vi "PH_Cam_BaseClass.ProcCases.vi"(0 "i ref in":refnum<vi>, 1 "selector":string, 2 "data":T1, 3 "call cluster":T2={"Object"="", "Selector"="", "CallType"=enum."synchronous", "Async Object"="", "Async Selector"="", "Data Descriptor"="", "Data"=[], "Error #"=0, "Expire"=0}, 5 "error in":errorcluster) -> (14 "i ref out":refnum<vi>, 17 "answer cluster":T2={"Object"="", "Selector"="", "CallType"=enum."synchronous", "Async Object"="", "Async Selector"="", "Data Descriptor"="", "Data"=[], "Error #"=0, "Expire"=0}, 19 "error out":errorcluster)   [LabVIEW 2014, in "PH_Cam_BaseClass.lvlib"]
doc: "This method is called by a process from within the default case in the event loop. The methods of a class that are linked to events will be called from THIS method. Add your code here."
uses:
  PH_Cam_BaseClass.lvlib
  CSCore/CSSystem/CoreDefs/CoreDefs.call_type.ctl
  CSCore/BaseProcess/BaseProcess.descriptor string definition.ctl
  CSCore/CSSystem/CoreDefs/CoreDefs.rawDataType.ctl
  CSCore/CSSystem/CoreLib/CoreLib.string 2 byte array.vi
  CSCore/CSSystem/CoreLib/CoreLib.byte array 2 string.vi
  CSCore/CSSystem/CoreLib/CoreLib.byte array 2 short.vi
  CSCore/CSSystem/CoreLib/CoreLib.byte array 2 double.vi
  CSCore/CSSystem/CoreLib/CoreLib.byte array 2 int.vi
  CSCore/CSSystem/CoreLib/CoreLib.lvlib
  CSCore/BaseProcess/BaseProcess.lvlib
  PH_Common/PH_Common.lvlib
  PH_PSDBWriter/PH_PSDBWriter.lvlib
panel:
  in  "EP":cluster{"Red":u8, "Green":u8, "Blue":u8}[](array[cluster])=[{"Red"=0, "Green"=255, "Blue"=0}, {"Red"=0, "Green"=245, "Blue"=0}, {"Red"=0, "Green"=235, "Blue"=0}, {"Red"=0, "Green"=225, "Blue"=0}, {"Red"=0, "Green"=215, "Blue"=0}, {"Red"=0, "Green"=205, "Blue"=0}, {"Red"=0, "Green"=195, "Blue"=0}, {"Red"=0, "Green"=185, "Blue"=0}, {"Red"=0, "Green"=175, "Blue"=0}, {"Red"=0, "Green"=165, "Blue"=0}, {"Red"=10, "Green"=10, "Blue"=10}, {"Red"=11, "Green"=11, "Blue"=11}, {"Red"=12, "Green"=12, "Blue"=12}, {"Red"=13, "Green"=13, "Blue"=13}, {"Red"=14, "Green"=14, "Blue"=14}, {"Red"=15, "Green"=15, "Blue"=15}, {"Red"=16, "Green"=16, "Blue"=16}, {"Red"=17, "Green"=17, "Blue"=17}, {"Red"=18, "Green"=18, "Blue"=18}, {"Red"=19, "Green"=19, "Blue"=19}, {"Red"=20, "Green"=20, "Blue"=20}, {"Red"=21, "Green"=21, "Blue"=21}, {"Red"=22, "Green"=22, "Blue"=22}, {"Red"=23, "Green"=23, "Blue"=23}, {"Red"=24, "Green"=24, "Blue"=24}, {"Red"=25, "Green"=25, "Blue"=25}, {"Red"=26, "Green"=26, "Blue"=26}, {"Red"=27, "Green"=27, "Blue"=27}, {"Red"=28, "Green"=28, "Blue"=28}, {"Red"=29, "Green"=29, "Blue"=29}, {"Red"=30, "Green"=30, "Blue"=30}, {"Red"=31, "Green"=31, "Blue"=31}, {"Red"=32, "Green"=32, "Blue"=32}, {"Red"=33, "Green"=33, "Blue"=33}, {"Red"=34, "Green"=34, "Blue"=34}, {"Red"=35, "Green"=35, "Blue"=35}, {"Red"=36, "Green"=36, "Blue"=36}, {"Red"=37, "Green"=37, "Blue"=37}, {"Red"=38, "Green"=38, "Blue"=38}, {"Red"=39, "Green"=39, "Blue"=39}, {"Red"=40, "Green"=40, "Blue"=40}, {"Red"=41, "Green"=41, "Blue"=41}, {"Red"=42, "Green"=42, "Blue"=42}, {"Red"=43, "Green"=43, "Blue"=43}, {"Red"=44, "Green"=44, "Blue"=44}, {"Red"=45, "Green"=45, "Blue"=45}, {"Red"=46, "Green"=46, "Blue"=46}, {"Red"=47, "Green"=47, "Blue"=47}, {"Red"=48, "Green"=48, "Blue"=48}, {"Red"=49, "Green"=49, "Blue"=49}, {"Red"=50, "Green"=50, "Blue"=50}, {"Red"=51, "Green"=51, "Blue"=51}, {"Red"=52, "Green"=52, "Blue"=52}, {"Red"=53, "Green"=53, "Blue"=53}, {"Red"=54, "Green"=54, "Blue"=54}, {"Red"=55, "Green"=55, "Blue"=55}, {"Red"=56, "Green"=56, "Blue"=56}, {"Red"=57, "Green"=57, "Blue"=57}, {"Red"=58, "Green"=58, "Blue"=58}, {"Red"=59, "Green"=59, "Blue"=59}, {"Red"=60, "Green"=60, "Blue"=60}, {"Red"=61, "Green"=61, "Blue"=61}, {"Red"=62, "Green"=62, "Blue"=62}, {"Red"=63, "Green"=63, "Blue"=63}, {"Red"=64, "Green"=64, "Blue"=64}, {"Red"=65, "Green"=65, "Blue"=65}, {"Red"=66, "Green"=66, "Blue"=66}, {"Red"=67, "Green"=67, "Blue"=67}, {"Red"=68, "Green"=68, "Blue"=68}, {"Red"=69, "Green"=69, "Blue"=69}, {"Red"=70, "Green"=70, "Blue"=70}, {"Red"=71, "Green"=71, "Blue"=71}, {"Red"=72, "Green"=72, "Blue"=72}, {"Red"=73, "Green"=73, "Blue"=73}, {"Red"=74, "Green"=74, "Blue"=74}, {"Red"=75, "Green"=75, "Blue"=75}, {"Red"=76, "Green"=76, "Blue"=76}, {"Red"=77, "Green"=77, "Blue"=77}, {"Red"=78, "Green"=78, "Blue"=78}, {"Red"=79, "Green"=79, "Blue"=79}, {"Red"=80, "Green"=80, "Blue"=80}, {"Red"=81, "Green"=81, "Blue"=81}, {"Red"=82, "Green"=82, "Blue"=82}, {"Red"=83, "Green"=83, "Blue"=83}, {"Red"=84, "Green"=84, "Blue"=84}, {"Red"=85, "Green"=85, "Blue"=85}, {"Red"=86, "Green"=86, "Blue"=86}, {"Red"=87, "Green"=87, "Blue"=87}, {"Red"=88, "Green"=88, "Blue"=88}, {"Red"=89, "Green"=89, "Blue"=89}, {"Red"=90, "Green"=90, "Blue"=90}, {"Red"=91, "Green"=91, "Blue"=91}, {"Red"=92, "Green"=92, "Blue"=92}, {"Red"=93, "Green"=93, "Blue"=93}, {"Red"=94, "Green"=94, "Blue"=94}, {"Red"=95, "Green"=95, "Blue"=95}, {"Red"=96, "Green"=96, "Blue"=96}, {"Red"=97, "Green"=97, "Blue"=97}, {"Red"=98, "Green"=98, "Blue"=98}, {"Red"=99, "Green"=99, "Blue"=99}, {"Red"=100, "Green"=100, "Blue"=100}, {"Red"=101, "Green"=101, "Blue"=101}, {"Red"=102, "Green"=102, "Blue"=102}, {"Red"=103, "Green"=103, "Blue"=103}, {"Red"=104, "Green"=104, "Blue"=104}, {"Red"=105, "Green"=105, "Blue"=105}, {"Red"=106, "Green"=106, "Blue"=106}, {"Red"=107, "Green"=107, "Blue"=107}, {"Red"=108, "Green"=108, "Blue"=108}, {"Red"=109, "Green"=109, "Blue"=109}, {"Red"=110, "Green"=110, "Blue"=110}, {"Red"=111, "Green"=111, "Blue"=111}, {"Red"=112, "Green"=112, "Blue"=112}, {"Red"=113, "Green"=113, "Blue"=113}, {"Red"=114, "Green"=114, "Blue"=114}, {"Red"=115, "Green"=115, "Blue"=115}, {"Red"=116, "Green"=116, "Blue"=116}, {"Red"=117, "Green"=117, "Blue"=117}, {"Red"=118, "Green"=118, "Blue"=118}, {"Red"=119, "Green"=119, "Blue"=119}, {"Red"=120, "Green"=120, "Blue"=120}, {"Red"=121, "Green"=121, "Blue"=121}, {"Red"=122, "Green"=122, "Blue"=122}, {"Red"=123, "Green"=123, "Blue"=123}, {"Red"=124, "Green"=124, "Blue"=124}, {"Red"=125, "Green"=125, "Blue"=125}, {"Red"=126, "Green"=126, "Blue"=126}, {"Red"=127, "Green"=127, "Blue"=127}, {"Red"=128, "Green"=128, "Blue"=128}, {"Red"=129, "Green"=129, "Blue"=129}, {"Red"=130, "Green"=130, "Blue"=130}, {"Red"=131, "Green"=131, "Blue"=131}, {"Red"=132, "Green"=132, "Blue"=132}, {"Red"=133, "Green"=133, "Blue"=133}, {"Red"=134, "Green"=134, "Blue"=134}, {"Red"=135, "Green"=135, "Blue"=135}, {"Red"=136, "Green"=136, "Blue"=136}, {"Red"=137, "Green"=137, "Blue"=137}, {"Red"=138, "Green"=138, "Blue"=138}, {"Red"=139, "Green"=139, "Blue"=139}, {"Red"=140, "Green"=140, "Blue"=140}, {"Red"=141, "Green"=141, "Blue"=141}, {"Red"=142, "Green"=142, "Blue"=142}, {"Red"=143, "Green"=143, "Blue"=143}, {"Red"=144, "Green"=144, "Blue"=144}, {"Red"=145, "Green"=145, "Blue"=145}, {"Red"=146, "Green"=146, "Blue"=146}, {"Red"=147, "Green"=147, "Blue"=147}, {"Red"=148, "Green"=148, "Blue"=148}, {"Red"=149, "Green"=149, "Blue"=149}, {"Red"=150, "Green"=150, "Blue"=150}, {"Red"=151, "Green"=151, "Blue"=151}, {"Red"=152, "Green"=152, "Blue"=152}, {"Red"=153, "Green"=153, "Blue"=153}, {"Red"=154, "Green"=154, "Blue"=154}, {"Red"=155, "Green"=155, "Blue"=155}, {"Red"=156, "Green"=156, "Blue"=156}, {"Red"=157, "Green"=157, "Blue"=157}, {"Red"=158, "Green"=158, "Blue"=158}, {"Red"=159, "Green"=159, "Blue"=159}, {"Red"=160, "Green"=160, "Blue"=160}, {"Red"=161, "Green"=161, "Blue"=161}, {"Red"=162, "Green"=162, "Blue"=162}, {"Red"=163, "Green"=163, "Blue"=163}, {"Red"=164, "Green"=164, "Blue"=164}, {"Red"=165, "Green"=165, "Blue"=165}, {"Red"=166, "Green"=166, "Blue"=166}, {"Red"=167, "Green"=167, "Blue"=167}, {"Red"=168, "Green"=168, "Blue"=168}, {"Red"=169, "Green"=169, "Blue"=169}, {"Red"=170, "Green"=170, "Blue"=170}, {"Red"=171, "Green"=171, "Blue"=171}, {"Red"=172, "Green"=172, "Blue"=172}, {"Red"=173, "Green"=173, "Blue"=173}, {"Red"=174, "Green"=174, "Blue"=174}, {"Red"=175, "Green"=175, "Blue"=175}, {"Red"=176, "Green"=176, "Blue"=176}, {"Red"=177, "Green"=177, "Blue"=177}, {"Red"=178, "Green"=178, "Blue"=178}, {"Red"=179, "Green"=179, "Blue"=179}, {"Red"=180, "Green"=180, "Blue"=180}, {"Red"=181, "Green"=181, "Blue"=181}, {"Red"=182, "Green"=182, "Blue"=182}, {"Red"=183, "Green"=183, "Blue"=183}, {"Red"=184, "Green"=184, "Blue"=184}, {"Red"=185, "Green"=185, "Blue"=185}, {"Red"=186, "Green"=186, "Blue"=186}, {"Red"=187, "Green"=187, "Blue"=187}, {"Red"=188, "Green"=188, "Blue"=188}, {"Red"=189, "Green"=189, "Blue"=189}, {"Red"=190, "Green"=190, "Blue"=190}, {"Red"=191, "Green"=191, "Blue"=191}, {"Red"=192, "Green"=192, "Blue"=192}, {"Red"=193, "Green"=193, "Blue"=193}, {"Red"=194, "Green"=194, "Blue"=194}, {"Red"=195, "Green"=195, "Blue"=195}, {"Red"=196, "Green"=196, "Blue"=196}, {"Red"=197, "Green"=197, "Blue"=197}, {"Red"=198, "Green"=198, "Blue"=198}, {"Red"=199, "Green"=199, "Blue"=199}, {"Red"=200, "Green"=200, "Blue"=200}, {"Red"=201, "Green"=201, "Blue"=201}, {"Red"=202, "Green"=202, "Blue"=202}, {"Red"=203, "Green"=203, "Blue"=203}, {"Red"=204, "Green"=204, "Blue"=204}, {"Red"=205, "Green"=205, "Blue"=205}, {"Red"=206, "Green"=206, "Blue"=206}, {"Red"=207, "Green"=207, "Blue"=207}, {"Red"=208, "Green"=208, "Blue"=208}, {"Red"=209, "Green"=209, "Blue"=209}, {"Red"=210, "Green"=210, "Blue"=210}, {"Red"=211, "Green"=211, "Blue"=211}, {"Red"=212, "Green"=212, "Blue"=212}, {"Red"=213, "Green"=213, "Blue"=213}, {"Red"=214, "Green"=214, "Blue"=214}, {"Red"=215, "Green"=215, "Blue"=215}, {"Red"=216, "Green"=216, "Blue"=216}, {"Red"=217, "Green"=217, "Blue"=217}, {"Red"=218, "Green"=218, "Blue"=218}, {"Red"=219, "Green"=219, "Blue"=219}, {"Red"=220, "Green"=220, "Blue"=220}, {"Red"=221, "Green"=221, "Blue"=221}, {"Red"=222, "Green"=222, "Blue"=222}, {"Red"=223, "Green"=223, "Blue"=223}, {"Red"=224, "Green"=224, "Blue"=224}, {"Red"=225, "Green"=225, "Blue"=225}, {"Red"=226, "Green"=226, "Blue"=226}, {"Red"=227, "Green"=227, "Blue"=227}, {"Red"=228, "Green"=228, "Blue"=228}, {"Red"=229, "Green"=229, "Blue"=229}, {"Red"=230, "Green"=230, "Blue"=230}, {"Red"=231, "Green"=231, "Blue"=231}, {"Red"=232, "Green"=232, "Blue"=232}, {"Red"=233, "Green"=233, "Blue"=233}, {"Red"=234, "Green"=234, "Blue"=234}, {"Red"=235, "Green"=235, "Blue"=235}, {"Red"=236, "Green"=236, "Blue"=236}, {"Red"=237, "Green"=237, "Blue"=237}, {"Red"=238, "Green"=238, "Blue"=238}, {"Red"=239, "Green"=239, "Blue"=239}, {"Red"=240, "Green"=240, "Blue"=240}, {"Red"=241, "Green"=241, "Blue"=241}, {"Red"=242, "Green"=242, "Blue"=242}, {"Red"=243, "Green"=243, "Blue"=243}, {"Red"=244, "Green"=244, "Blue"=244}, {"Red"=245, "Green"=245, "Blue"=245}, {"Red"=165, "Green"=0, "Blue"=0}, {"Red"=175, "Green"=0, "Blue"=0}, {"Red"=185, "Green"=0, "Blue"=0}, {"Red"=195, "Green"=0, "Blue"=0}, {"Red"=205, "Green"=0, "Blue"=0}, {"Red"=215, "Green"=0, "Blue"=0}, {"Red"=225, "Green"=0, "Blue"=0}, {"Red"=235, "Green"=0, "Blue"=0}, {"Red"=245, "Green"=0, "Blue"=0}, {"Red"=255, "Green"=0, "Blue"=0}]
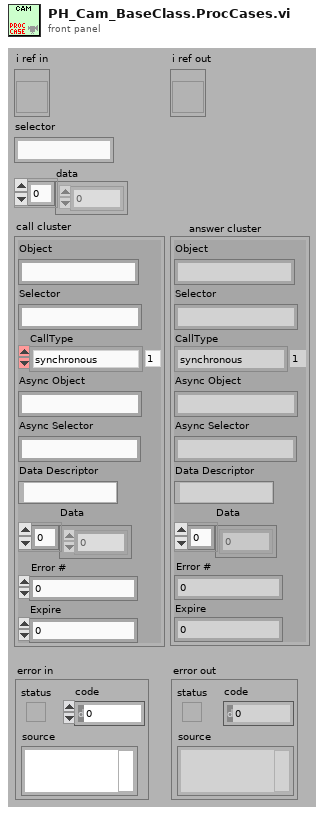
[diagram p1: front panel]
types:
  T1 = typedef "CoreDefs.rawDataType.ctl" = i8[]
  T2 = typedef "CoreDefs.call_type.ctl" = cluster{"Object":string, "Selector":string, "CallType":enum16{"simple", "synchronous", "asynchronous"}, "Async Object":string, "Async Selector":string, "Data Descriptor":T3, "Data":T1, "Error #":i32, "Expire":u32}
  T3 = typedef "BaseProcess.lvlib/BaseProcess.descriptor string definition.ctl" = string
  T4 = typedef "PH_Cam_BaseClass.lvlib/PH_Cam_BaseClass.i attribute.ctl" = cluster{"Gui Refs":T5, "Cam":cluster{"Source Notifier":refnum<notifier>, "Error":errorcluster, "Camera ID":string}, "Images":cluster{"Cam":T6, "Operation":T6, "PSDB":T6}, "Window Image":cluster{"Indicate Image":bool, "Window No.":i32, "Scale Facor":dbl, "Center Cross":bool, "Subtract Backgr":bool, "CoG":bool, "Color Palette":cluster{"Red":u8, "Green":u8, "Blue":u8}[], "Image On":bool}, "Default Prdc Int":i32, "Performance":cluster{"on":bool, "Timestamp Last Frame":i32}, "Histogram":cluster{"on":bool, "Mapping":bool}, "Save Image":cluster{"Save":bool, "File refnum":refnum<file>}, "Setting Service ID":i32, "Screen":cluster{"x-resolution":i16, "y-resolution":i16}, "On":bool, "Constructor finished":bool, "configured":bool}
  T5 = typedef "PH_Cam_BaseClass.lvlib/PH_Cam_BaseClass.GUI Refs.ctl" = cluster{"Frame Rate":refnum<vi>, "Get Frame Rate":refnum<vi>, "Show Image":refnum<vi>, "Get Histogram":refnum<vi>, "Mapping":refnum<vi>, "Histogram":refnum<vi>, "Center Cross":refnum<vi>, "Center of Gravity":refnum<vi>, "Scale Factor [%]":refnum<vi>, "Save Image":refnum<vi>, "Palette":refnum<vi>, "Subtract Background":refnum<vi>, "Cam Error":refnum<vi>, "On":refnum<vi>, "Cam List":refnum<vi>}
  T6 = typedef "IMAQ Image.ctl" = refnum<image>
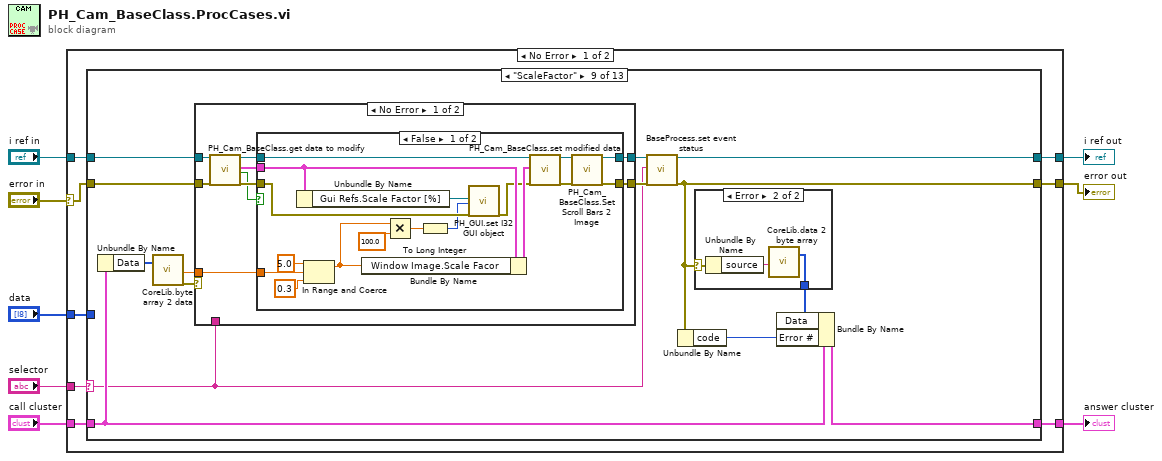
[diagram p0: block diagram]
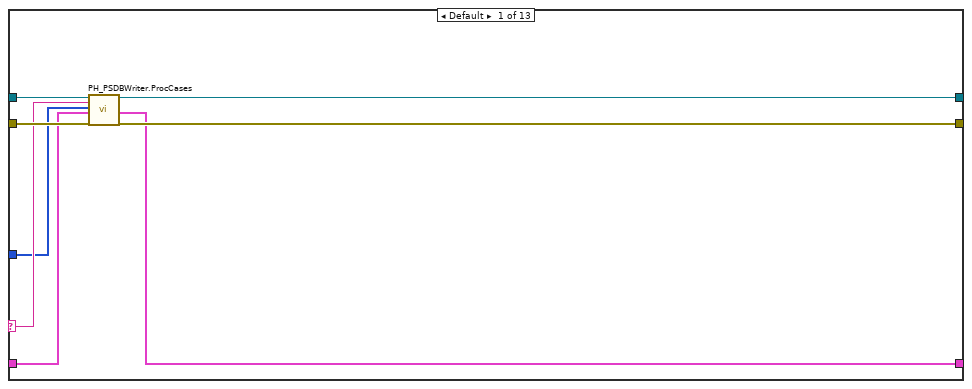
[diagram p2: hidden frame]
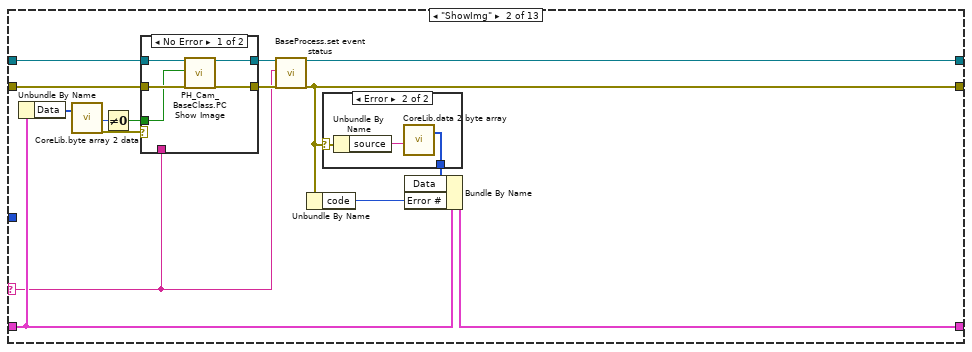
[diagram p3: hidden frame]
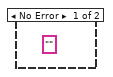
[diagram p4: hidden frame]
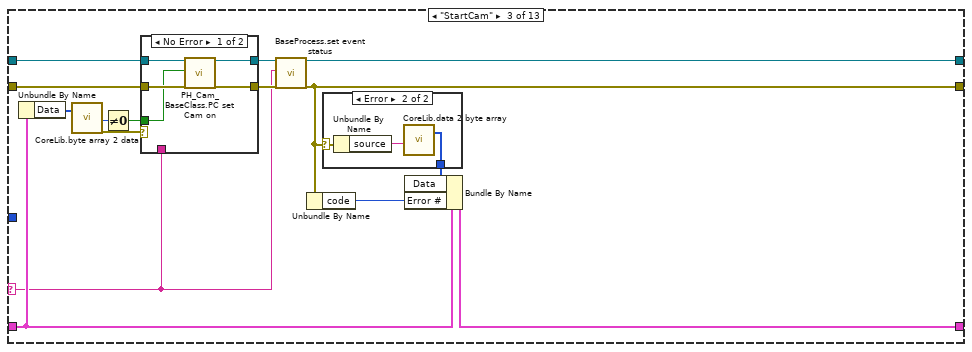
[diagram p6: hidden frame]
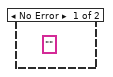
[diagram p7: hidden frame]
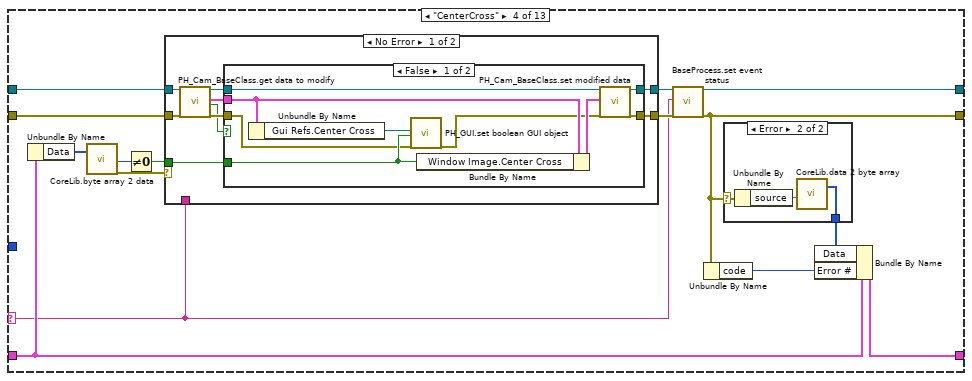
[diagram p9: hidden frame]
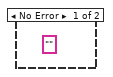
[diagram p10: hidden frame]
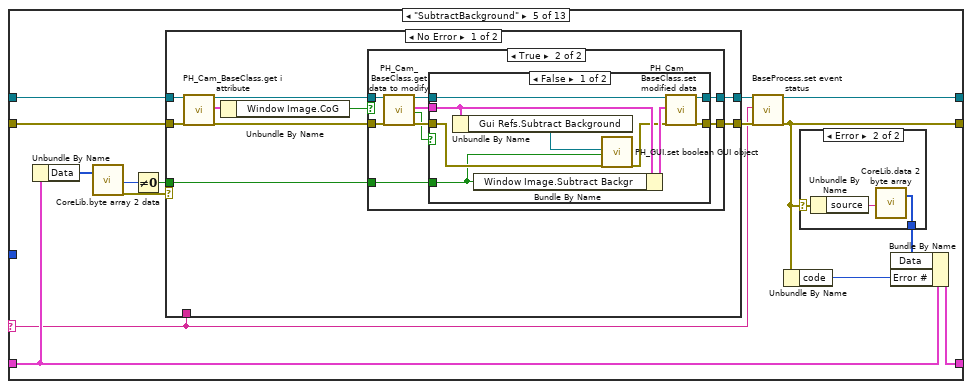
[diagram p13: hidden frame]
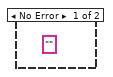
[diagram p14: hidden frame]
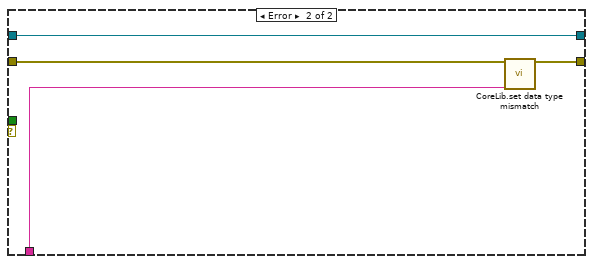
[diagram p17: hidden frame]
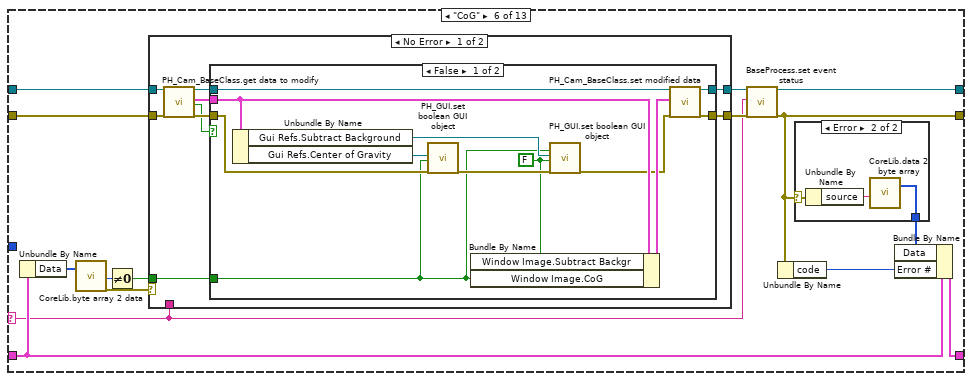
[diagram p18: hidden frame]
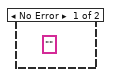
[diagram p19: hidden frame]
diagram:
  n1 = case shown="No Error" "error in" {
    selector: "error in" -> [w9 w553]
    tunnel: "selector" -> [w16 _]
    tunnel: [w15 w552] -> w7
    tunnel: "call cluster" -> [w14 w552]
    tunnel: "i ref in" -> [w13 w554]
    tunnel: [w12 w554] -> w4
    tunnel: [w11 w553] -> w3
    tunnel: "data" -> [w10 _]
    frame No Error {
      n2 = case shown="\"ScaleFactor\"" w16 {
        selector: w16 -> [w19 w31 w58 w85 w127 w180 w234 w283 w338 w388 w439 w492 w513]
        tunnel: w13 -> [w18 w39 w66 w93 w135 w188 w242 w291 w346 w396 w447 w500 w518]
        tunnel: [w24 w30 w57 w84 w126 w179 w233 w282 w337 w387 w438 w491 w523] -> w12
        tunnel: w14 -> [w20 w36 w63 w90 w132 w185 w239 w288 w343 w393 w444 w497 w516]
        tunnel: [w21 w35 w62 w89 w131 w184 w238 w287 w342 w392 w443 w496 w525] -> w15
        tunnel: w9 -> [w23 w38 w65 w92 w134 w187 w241 w290 w345 w395 w446 w499 w517]
        tunnel: [w22 w32 w59 w86 w128 w181 w235 w284 w339 w389 w440 w493 w524] -> w11
        tunnel: w10 -> [w17 _ _ _ _ _ _ _ _ _ _ _ _]
        frame Default {
          # "In the default case, always call the ProcCase method of the parent class"
          n3 = call "PH_PSDBWriter.ProcCases.vi"("i ref in"=w18, "selector"=w19, "Data"=w17, "call cluster"=w20, "error in"=w23) -> ("i ref out"=w24:refnum<vi>, "answer cluster"=w21:T2, "error out"=w22:errorcluster)  [unwired: 12 in]
        }
        frame "ShowImg" {
          n4 = Unbundle By Name(w36) -> ("Data"=w26:T1)
          n5 = call-poly "CoreLib.byte array 2 data.vi"("byteArray"=w26) -> ("i16"=w29:i16, "error out"=w28:errorcluster)  [unwired: 16 in, 1 out]
          n6 = Not Equal To 0?(x=w29) -> (x != 0?=w27:bool)
          n7 = case shown="No Error" w28 {
            tunnel: [w44 w51] -> w34
            tunnel: w39 -> [w46 w51]
            tunnel: w38 -> [w47 w50]
            tunnel: [w43 w49] -> w33
            tunnel: w31 -> [_ w48]
            tunnel: w27 -> [w45 _]
            frame No Error {
              n8 = call "PH_Cam_BaseClass.PC Show Image.vi"("i ref in"=w46, "Show Image"=w45, "error IO"=w47) -> ("i ref out"=w44:refnum<vi>, "error out"=w43:errorcluster)  [unwired: 15 in]
            }
            frame Error {
              n9 = call "CoreLib.set data type mismatch.vi"("error in (no error)"=w50, "error source"=w48) -> ("error out"=w49:errorcluster)  [unwired: 17 in]
            }
          }
          n10 = call "BaseProcess.set event status.vi"("i ref in"=w34, "EventStatus"=w31, "error in (no error)"=w33) -> ("i ref out"=w30:refnum<vi>, "error out"=w32:errorcluster)  [unwired: 14 in, 1 out]
          n11 = Unbundle By Name(w32) -> ("code"=w37:i32)
          n12 = case shown="Error" w32 {
            selector: w32 -> [_ w42]
            tunnel: [_ w40] -> w25
            frame No Error {
              (unwired) "" ("source")
            }
            frame Error {
              n13 = Unbundle By Name(w42) -> ("source"=w41:string)
              n14 = call-poly "CoreLib.data 2 byte array.vi"("string"=w41) -> ("byteArray out"=w40:T1)  [unwired: 18 in]
            }
          }
          n15 = Bundle By Name(cluster=w36, "Data"=w25, "Error #"=w37) -> (w35:T2)
        }
        frame "StartCam" {
          n16 = Unbundle By Name(w63) -> ("Data"=w53:T1)
          n17 = call-poly "CoreLib.byte array 2 data.vi"("byteArray"=w53) -> ("i16"=w56:i16, "error out"=w55:errorcluster)  [unwired: 16 in, 1 out]
          n18 = Not Equal To 0?(x=w56) -> (x != 0?=w54:bool)
          n19 = case shown="No Error" w55 {
            tunnel: [w71 w78] -> w61
            tunnel: w66 -> [w73 w78]
            tunnel: w65 -> [w74 w77]
            tunnel: [w70 w76] -> w60
            tunnel: w58 -> [_ w75]
            tunnel: w54 -> [w72 _]
            frame No Error {
              n20 = call "PH_Cam_BaseClass.PC set Cam on.vi"("i ref in"=w73, "Cam on"=w72, "error in (no error)"=w74) -> ("i ref out"=w71:refnum<vi>, "error out"=w70:errorcluster)  [unwired: 15 in]
            }
            frame Error {
              n21 = call "CoreLib.set data type mismatch.vi"("error in (no error)"=w77, "error source"=w75) -> ("error out"=w76:errorcluster)  [unwired: 17 in]
            }
          }
          n22 = call "BaseProcess.set event status.vi"("i ref in"=w61, "EventStatus"=w58, "error in (no error)"=w60) -> ("i ref out"=w57:refnum<vi>, "error out"=w59:errorcluster)  [unwired: 14 in, 1 out]
          n23 = Unbundle By Name(w59) -> ("code"=w64:i32)
          n24 = case shown="Error" w59 {
            selector: w59 -> [_ w69]
            tunnel: [_ w67] -> w52
            frame No Error {
              (unwired) "" ("source")
            }
            frame Error {
              n25 = Unbundle By Name(w69) -> ("source"=w68:string)
              n26 = call-poly "CoreLib.data 2 byte array.vi"("string"=w68) -> ("byteArray out"=w67:T1)  [unwired: 18 in]
            }
          }
          n27 = Bundle By Name(cluster=w63, "Data"=w52, "Error #"=w64) -> (w62:T2)
        }
        frame "CenterCross" {
          n28 = Unbundle By Name(w90) -> ("Data"=w80:T1)
          n29 = call-poly "CoreLib.byte array 2 data.vi"("byteArray"=w80) -> ("i16"=w83:i16, "error out"=w81:errorcluster)  [unwired: 16 in, 1 out]
          n30 = Not Equal To 0?(x=w83) -> (x != 0?=w82:bool)
          n31 = case shown="No Error" w81 {
            tunnel: [w100 w120] -> w88
            tunnel: w93 -> [w104 w120]
            tunnel: w92 -> [w105 w119]
            tunnel: [w102 w118] -> w87
            tunnel: w85 -> [_ w117]
            tunnel: w82 -> [w98 _]
            frame No Error {
              n32 = call "PH_Cam_BaseClass.get data to modify.vi"("i ref in"=w104, "error in (no error)"=w105) -> ("i ref out"=w101:refnum<vi>, "i attribute"=w99:T4, "timed out"=w97:bool, "error out"=w103:errorcluster)  [unwired: 14 in]
              n33 = case shown="False" w97 {
                tunnel: w103 -> [w107 w115]
                tunnel: [w114 w115] -> w102
                tunnel: w101 -> [w113 w116]
                tunnel: [w112 w116] -> w100
                tunnel: w99 -> [w110 _]
                tunnel: w98 -> [w108 _]
                frame False {
                  n34 = Unbundle By Name(w110) -> ("Gui Refs.Center Cross"=w109:refnum<vi>)
                  n35 = call "PH_GUI.set boolean GUI object.vi"("Boolean Knob GUI Ref"=w109, "Value"=w108, "error in (no error)"=w107) -> ("error out"=w106:errorcluster)  [unwired: 16 in]
                  n36 = Bundle By Name(cluster=w110, "Window Image.Center Cross"=w108) -> (w111:T4)
                  n37 = call "PH_Cam_BaseClass.set modified data.vi"("i ref in"=w113, "i attribute"=w111, "error in (no error)"=w106) -> ("i ref out"=w112:refnum<vi>, "error out"=w114:errorcluster)  [unwired: 15 in]
                }
                frame True {
                }
              }
            }
            frame Error {
              n38 = call "CoreLib.set data type mismatch.vi"("error in (no error)"=w119, "error source"=w117) -> ("error out"=w118:errorcluster)  [unwired: 17 in]
            }
          }
          n39 = call "BaseProcess.set event status.vi"("i ref in"=w88, "EventStatus"=w85, "error in (no error)"=w87) -> ("i ref out"=w84:refnum<vi>, "error out"=w86:errorcluster)  [unwired: 14 in, 1 out]
          n40 = Unbundle By Name(w86) -> ("code"=w91:i32)
          n41 = case shown="Error" w86 {
            selector: w86 -> [_ w96]
            tunnel: [_ w94] -> w79
            frame No Error {
              (unwired) "" ("source")
            }
            frame Error {
              n42 = Unbundle By Name(w96) -> ("source"=w95:string)
              n43 = call-poly "CoreLib.data 2 byte array.vi"("string"=w95) -> ("byteArray out"=w94:T1)  [unwired: 18 in]
            }
          }
          n44 = Bundle By Name(cluster=w90, "Data"=w79, "Error #"=w91) -> (w89:T2)
        }
        frame "SubtractBackground" {
          n45 = Unbundle By Name(w132) -> ("Data"=w122:T1)
          n46 = call-poly "CoreLib.byte array 2 data.vi"("byteArray"=w122) -> ("i16"=w125:i16, "error out"=w123:errorcluster)  [unwired: 16 in, 1 out]
          n47 = Not Equal To 0?(x=w125) -> (x != 0?=w124:bool)
          n48 = case shown="No Error" w123 {
            tunnel: [w145 w173] -> w130
            tunnel: w135 -> [w142 w173]
            tunnel: w134 -> [w147 w172]
            tunnel: [w146 w171] -> w129
            tunnel: w127 -> [_ w170]
            tunnel: w124 -> [w144 _]
            frame No Error {
              n49 = call "PH_Cam_BaseClass.get i attribute.vi"("i ref in"=w142, "error in (no error)"=w147) -> ("i ref out"=w141:refnum<vi>, "i attribute"=w140:T4, "error out"=w143:errorcluster)  [unwired: 15 in]
              n50 = Unbundle By Name(w140) -> ("Window Image.CoG"=w139:bool)
              n51 = case shown="True" w139 {
                tunnel: [w148 w157] -> w146
                tunnel: [w149 w155] -> w145
                tunnel: w144 -> [_ w153]
                tunnel: w143 -> [w148 w151]
                tunnel: w141 -> [w149 w150]
                frame False {
                }
                frame True {
                  n52 = call "PH_Cam_BaseClass.get data to modify.vi"("i ref in"=w150, "error in (no error)"=w151) -> ("i ref out"=w156:refnum<vi>, "i attribute"=w154:T4, "timed out"=w152:bool, "error out"=w158:errorcluster)  [unwired: 14 in]
                  n53 = case shown="False" w152 {
                    tunnel: w158 -> [w162 w168]
                    tunnel: [w167 w168] -> w157
                    tunnel: w156 -> [w166 w169]
                    tunnel: [w165 w169] -> w155
                    tunnel: w154 -> [w163 _]
                    tunnel: w153 -> [w161 _]
                    frame False {
                      n54 = Unbundle By Name(w163) -> ("Gui Refs.Subtract Background"=w160:refnum<vi>)
                      n55 = Bundle By Name(cluster=w163, "Window Image.Subtract Backgr"=w161) -> (w164:T4)
                      n56 = call "PH_GUI.set boolean GUI object.vi"("Boolean Knob GUI Ref"=w160, "Value"=w161, "error in (no error)"=w162) -> ("error out"=w159:errorcluster)  [unwired: 16 in]
                      n57 = call "PH_Cam_BaseClass.set modified data.vi"("i ref in"=w166, "i attribute"=w164, "error in (no error)"=w159) -> ("i ref out"=w165:refnum<vi>, "error out"=w167:errorcluster)  [unwired: 15 in]
                    }
                    frame True {
                    }
                  }
                }
              }
            }
            frame Error {
              n58 = call "CoreLib.set data type mismatch.vi"("error in (no error)"=w172, "error source"=w170) -> ("error out"=w171:errorcluster)  [unwired: 17 in]
            }
          }
          n59 = call "BaseProcess.set event status.vi"("i ref in"=w130, "EventStatus"=w127, "error in (no error)"=w129) -> ("i ref out"=w126:refnum<vi>, "error out"=w128:errorcluster)  [unwired: 14 in, 1 out]
          n60 = Unbundle By Name(w128) -> ("code"=w133:i32)
          n61 = case shown="Error" w128 {
            selector: w128 -> [_ w138]
            tunnel: [_ w136] -> w121
            frame No Error {
              (unwired) "" ("source")
            }
            frame Error {
              n62 = Unbundle By Name(w138) -> ("source"=w137:string)
              n63 = call-poly "CoreLib.data 2 byte array.vi"("string"=w137) -> ("byteArray out"=w136:T1)  [unwired: 18 in]
            }
          }
          n64 = Bundle By Name(cluster=w132, "Data"=w121, "Error #"=w133) -> (w131:T2)
        }
        frame "CoG" {
          n65 = Unbundle By Name(w185) -> ("Data"=w175:T1)
          n66 = call-poly "CoreLib.byte array 2 data.vi"("byteArray"=w175) -> ("i16"=w178:i16, "error out"=w176:errorcluster)  [unwired: 16 in, 1 out]
          n67 = Not Equal To 0?(x=w178) -> (x != 0?=w177:bool)
          n68 = case shown="No Error" w176 {
            tunnel: [w195 w218] -> w183
            tunnel: w188 -> [w199 w218]
            tunnel: w187 -> [w200 w217]
            tunnel: [w197 w216] -> w182
            tunnel: w180 -> [_ w215]
            tunnel: w177 -> [w193 _]
            frame No Error {
              n69 = call "PH_Cam_BaseClass.get data to modify.vi"("i ref in"=w199, "error in (no error)"=w200) -> ("i ref out"=w196:refnum<vi>, "i attribute"=w194:T4, "timed out"=w192:bool, "error out"=w198:errorcluster)  [unwired: 14 in]
              n70 = case shown="False" w192 {
                tunnel: w198 -> [w206 w213]
                tunnel: [w212 w213] -> w197
                tunnel: w196 -> [w211 w214]
                tunnel: [w210 w214] -> w195
                tunnel: w194 -> [w208 _]
                tunnel: w193 -> [w202 _]
                frame False {
                  w201 = FALSE ("Value")
                  n71 = Unbundle By Name(w208) -> ("Gui Refs.Subtract Background"=w203:refnum<vi>, "Gui Refs.Center of Gravity"=w207:refnum<vi>)
                  n72 = call "PH_GUI.set boolean GUI object.vi"("Boolean Knob GUI Ref"=w207, "Value"=w202, "error in (no error)"=w206) -> ("error out"=w205:errorcluster)  [unwired: 16 in]
                  n73 = Bundle By Name(cluster=w208, "Window Image.Subtract Backgr"=w201, "Window Image.CoG"=w202) -> (w209:T4)
                  n74 = call "PH_GUI.set boolean GUI object.vi"("Visible (true)"=w202, "Boolean Knob GUI Ref"=w203, "Value"=w201, "error in (no error)"=w205) -> ("error out"=w204:errorcluster)  [unwired: 15 in]
                  n75 = call "PH_Cam_BaseClass.set modified data.vi"("i ref in"=w211, "i attribute"=w209, "error in (no error)"=w204) -> ("i ref out"=w210:refnum<vi>, "error out"=w212:errorcluster)  [unwired: 15 in]
                }
                frame True {
                }
              }
            }
            frame Error {
              n76 = call "CoreLib.set data type mismatch.vi"("error in (no error)"=w217, "error source"=w215) -> ("error out"=w216:errorcluster)  [unwired: 17 in]
            }
          }
          n77 = call "BaseProcess.set event status.vi"("i ref in"=w183, "EventStatus"=w180, "error in (no error)"=w182) -> ("i ref out"=w179:refnum<vi>, "error out"=w181:errorcluster)  [unwired: 14 in, 1 out]
          n78 = Unbundle By Name(w181) -> ("code"=w186:i32)
          n79 = case shown="Error" w181 {
            selector: w181 -> [_ w191]
            tunnel: [_ w189] -> w174
            frame No Error {
              (unwired) "" ("source")
            }
            frame Error {
              n80 = Unbundle By Name(w191) -> ("source"=w190:string)
              n81 = call-poly "CoreLib.data 2 byte array.vi"("string"=w190) -> ("byteArray out"=w189:T1)  [unwired: 18 in]
            }
          }
          n82 = Bundle By Name(cluster=w185, "Data"=w174, "Error #"=w186) -> (w184:T2)
        }
        frame "SaveImg" {
          n83 = Unbundle By Name(w239) -> ("Data"=w227:T1)
          n84 = call-poly "CoreLib.byte array 2 data.vi"("byteArray"=w227) -> ("byteArray out"=w226:T1, "i16"=w229:i16, "error out"=w225:errorcluster)  [unwired: 16 in]
          n85 = Not Equal To 0?(x=w229) -> (x != 0?=w228:bool)
          n86 = call-poly "CoreLib.byte array 2 data.vi"("byteArray"=w226, "error in (no error)"=w225) -> ("string"=w224:string, "error out"=w222:errorcluster)  [unwired: 15 in, 1 out]
          n87 = Unflatten From String(type=refnum<file> refnum ("File refnum"), binary string=w224) -> (value=w231:refnum<file>, error out=w220:errorcluster)  [unwired: 3 in, 1 out]
          n88 = Unbundle By Name(w220) -> ("status"=w219:bool)
          n89 = Unbundle By Name(w222) -> ("status"=w221:bool)
          n90 = Or(x=w219, y=w221) -> (x .or. y?=w223:bool)
          n91 = case shown="False" w223 {
            tunnel: [w250 w277] -> w237
            tunnel: w242 -> [w256 w277]
            tunnel: w241 -> [w257 w276]
            tunnel: [w248 w275] -> w236
            tunnel: w234 -> [_ w274]
            tunnel: w228 -> [w246 _]
            tunnel: w231 -> [w255 _]
            frame False {
              n92 = call "PH_Cam_BaseClass.get data to modify.vi"("i ref in"=w256, "error in (no error)"=w257) -> ("i ref out"=w253:refnum<vi>, "i attribute"=w252:T4, "timed out"=w251:bool, "error out"=w254:errorcluster)  [unwired: 14 in]
              n93 = case shown="False" w251 {
                tunnel: w254 -> [w266 w272]
                tunnel: [w271 w272] -> w247
                tunnel: w253 -> [w270 w273]
                tunnel: [w269 w273] -> w249
                tunnel: w252 -> [w267 _]
                tunnel: w255 -> [w265 _]
                frame False {
                  n94 = Bundle By Name(cluster=w267, "Save Image.Save"=TRUE, "Save Image.File refnum"=w265) -> (w268:T4)
                  n95 = call "PH_Cam_BaseClass.set modified data.vi"("i ref in"=w270, "i attribute"=w268, "error in (no error)"=w266) -> ("i ref out"=w269:refnum<vi>, "error out"=w271:errorcluster)  [unwired: 15 in]
                }
                frame True {
                }
              }
              n96 = case shown="False" w246 {
                tunnel: [w261 w263] -> w250
                tunnel: w249 -> [w258 w263]
                tunnel: [w260 w262] -> w248
                tunnel: w247 -> [w259 w262]
                frame False {
                  n97 = call "PH_Cam_BaseClass.save Image.vi"("i ref in"=w258, "error in (no error)"=w259) -> ("i ref out"=w261:refnum<vi>, "error out"=w260:errorcluster)  [unwired: 16 in]
                }
                frame True {
                }
              }
            }
            frame True {
              n98 = call "CoreLib.set data type mismatch.vi"("error in (no error)"=w276, "error source"=w274) -> ("error out"=w275:errorcluster)  [unwired: 17 in]
            }
          }
          n99 = call "BaseProcess.set event status.vi"("i ref in"=w237, "EventStatus"=w234, "error in (no error)"=w236) -> ("i ref out"=w233:refnum<vi>, "error out"=w235:errorcluster)  [unwired: 14 in, 1 out]
          n100 = Unbundle By Name(w235) -> ("code"=w240:i32)
          n101 = case shown="Error" w235 {
            selector: w235 -> [_ w245]
            tunnel: [_ w243] -> w230
            frame No Error {
              (unwired) "" ("source")
            }
            frame Error {
              n102 = Unbundle By Name(w245) -> ("source"=w244:string)
              n103 = call-poly "CoreLib.data 2 byte array.vi"("string"=w244) -> ("byteArray out"=w243:T1)  [unwired: 18 in]
            }
          }
          n104 = Bundle By Name(cluster=w239, "Data"=w230, "Error #"=w240) -> (w238:T2)
        }
        frame "SetPalette" {
          n105 = Unbundle By Name(w288) -> ("Data"=w281:T1)
          n106 = call-poly "CoreLib.byte array 2 data.vi"("byteArray"=w281) -> ("i32"=w280:i32, "error out"=w279:errorcluster)  [unwired: 16 in, 1 out]
          n107 = case shown="No Error" w279 {
            tunnel: [w298 w332] -> w286
            tunnel: w291 -> [w302 w332]
            tunnel: w290 -> [w303 w331]
            tunnel: [w300 w330] -> w285
            tunnel: w283 -> [_ w329]
            tunnel: w280 -> [w296 _]
            frame No Error {
              n108 = call "PH_Cam_BaseClass.get data to modify.vi"("i ref in"=w302, "error in (no error)"=w303) -> ("i ref out"=w299:refnum<vi>, "i attribute"=w297:T4, "timed out"=w295:bool, "error out"=w301:errorcluster)  [unwired: 14 in]
              n109 = case shown="False" w295 {
                tunnel: w301 -> [w307 w327]
                tunnel: [w315 w327] -> w300
                tunnel: w299 -> [w314 w328]
                tunnel: [w313 w328] -> w298
                tunnel: w297 -> [w311 _]
                tunnel: w296 -> [w308 _]
                frame False {
                  n110 = Unbundle By Name(w311) -> ("Gui Refs.Palette"=w304:refnum<vi>)
                  n111 = case shown="0..4" w308 {
                    selector: w308 -> [w316 _]
                    tunnel: w307 -> [w319 w321]
                    tunnel: [w318 w321] -> w306
                    tunnel: [w317 "EP"] -> w305
                    frame 0..4 {
                      n112 = call "IMAQ GetPalette"("Palette Number (gray)"=w316, "error in (no error)"=w319) -> ("Color Palette"=w317:cluster{"Red":u8, "Green":u8, "Blue":u8}[], "error out"=w318:errorcluster)  [unwired: 3 in]
                    }
                    frame 5, Default {
                    }
                  }
                  n113 = Not A Number/Path/Refnum?(number/path/refnum=w304) -> (NaN/Path/Refnum?=w310:bool)
                  n114 = Bundle By Name(cluster=w311, "Window Image.Color Palette"=w305) -> (w312:T4)
                  n115 = case shown="False" w310 {
                    tunnel: w306 -> [w325 w326]
                    tunnel: [w324 w326] -> w309
                    tunnel: w304 -> [w323 _]
                    tunnel: w308 -> [w322 _]
                    frame False {
                      n116 = property class="Ring (strict)"(reference=w323, error in=w325, "Value"=w322) -> (error out=w324:errorcluster)  [unwired: 1 out]
                    }
                    frame True {
                    }
                  }
                  n117 = call "PH_Cam_BaseClass.set modified data.vi"("i ref in"=w314, "i attribute"=w312, "error in (no error)"=w309) -> ("i ref out"=w313:refnum<vi>, "error out"=w315:errorcluster)  [unwired: 15 in]
                }
                frame True {
                }
              }
            }
            frame Error {
              n118 = call "CoreLib.set data type mismatch.vi"("error in (no error)"=w331, "error source"=w329) -> ("error out"=w330:errorcluster)  [unwired: 17 in]
            }
          }
          n119 = call "BaseProcess.set event status.vi"("i ref in"=w286, "EventStatus"=w283, "error in (no error)"=w285) -> ("i ref out"=w282:refnum<vi>, "error out"=w284:errorcluster)  [unwired: 14 in, 1 out]
          n120 = Unbundle By Name(w284) -> ("code"=w289:i32)
          n121 = case shown="Error" w284 {
            selector: w284 -> [_ w294]
            tunnel: [_ w292] -> w278
            frame No Error {
            }
            frame Error {
              n122 = Unbundle By Name(w294) -> ("source"=w293:string)
              n123 = call-poly "CoreLib.data 2 byte array.vi"("string"=w293) -> ("byteArray out"=w292:T1)  [unwired: 18 in]
            }
          }
          n124 = Bundle By Name(cluster=w288, "Data"=w278, "Error #"=w289) -> (w287:T2)
        }
        frame "ScaleFactor" {
          n125 = Unbundle By Name(w343) -> ("Data"=w336:T1)
          n126 = call-poly "CoreLib.byte array 2 data.vi"("byteArray"=w336) -> ("d64"=w335:dbl, "error out"=w334:errorcluster)  [unwired: 16 in, 1 out]
          n127 = case shown="No Error" w334 {
            tunnel: [w350 w381] -> w341
            tunnel: w346 -> [w357 w381]
            tunnel: w345 -> [w358 w380]
            tunnel: [w351 w379] -> w340
            tunnel: w338 -> [_ w378]
            tunnel: w335 -> [w353 _]
            frame No Error {
              n128 = call "PH_Cam_BaseClass.get data to modify.vi"("i ref in"=w357, "error in (no error)"=w358) -> ("i ref out"=w355:refnum<vi>, "i attribute"=w354:T4, "timed out"=w352:bool, "error out"=w356:errorcluster)  [unwired: 14 in]
              n129 = case shown="False" w352 {
                tunnel: w356 -> [w372 w376]
                tunnel: [w359 w376] -> w351
                tunnel: w355 -> [w375 w377]
                tunnel: [w360 w377] -> w350
                tunnel: w354 -> [w373 _]
                tunnel: w353 -> [w368 _]
                frame False {
                  n130 = Unbundle By Name(w373) -> ("Gui Refs.Scale Factor [%]"=w364:refnum<vi>)
                  n131 = In Range and Coerce(upper limit=5.0, x=w368, lower limit=0.3) -> (coerced(x)=w369:dbl)  [unwired: 1 out]
                  n132 = Bundle By Name(cluster=w373, "Window Image.Scale Facor"=w369) -> (w374:T4)
                  n133 = Multiply(x=w369, y=100.0) -> (x*y=w370:dbl)
                  n134 = To Long Integer(number=w370) -> (32bit integer=w363:i32)
                  n135 = call "PH_GUI.set I32 GUI object.vi"("I32 GUI Ref"=w364, "value"=w363, "error in (no error)"=w372) -> ("error out"=w365:errorcluster)  [unwired: 16 in]
                  n136 = call "PH_Cam_BaseClass.set modified data.vi"("i ref in"=w375, "i attribute"=w374, "error in (no error)"=w365) -> ("i ref out"=w361:refnum<vi>, "error out"=w362:errorcluster)  [unwired: 15 in]
                  n137 = call "PH_Cam_BaseClass.Set Scroll Bars 2 Image.vi"("i ref in"=w361, "error in (no error)"=w362) -> ("i ref out"=w360:refnum<vi>, "error out"=w359:errorcluster)  [unwired: 16 in]
                }
                frame True {
                }
              }
            }
            frame Error {
              n138 = call "CoreLib.set data type mismatch.vi"("error in (no error)"=w380, "error source"=w378) -> ("error out"=w379:errorcluster)  [unwired: 17 in]
            }
          }
          n139 = call "BaseProcess.set event status.vi"("i ref in"=w341, "EventStatus"=w338, "error in (no error)"=w340) -> ("i ref out"=w337:refnum<vi>, "error out"=w339:errorcluster)  [unwired: 14 in, 1 out]
          n140 = Unbundle By Name(w339) -> ("code"=w344:i32)
          n141 = case shown="Error" w339 {
            selector: w339 -> [_ w349]
            tunnel: [_ w347] -> w333
            frame No Error {
              (unwired) "" ("source")
            }
            frame Error {
              n142 = Unbundle By Name(w349) -> ("source"=w348:string)
              n143 = call-poly "CoreLib.data 2 byte array.vi"("string"=w348) -> ("byteArray out"=w347:T1)  [unwired: 18 in]
            }
          }
          n144 = Bundle By Name(cluster=w343, "Data"=w333, "Error #"=w344) -> (w342:T2)
        }
        frame "GetHistogram" {
          n145 = Unbundle By Name(w393) -> ("Data"=w385:T1)
          n146 = call-poly "CoreLib.byte array 2 data.vi"("byteArray"=w385) -> ("i16"=w386:i16, "error out"=w383:errorcluster)  [unwired: 16 in, 1 out]
          n147 = Not Equal To 0?(x=w386) -> (x != 0?=w384:bool)
          n148 = case shown="No Error" w383 {
            tunnel: [w403 w432] -> w391
            tunnel: w396 -> [w407 w432]
            tunnel: w395 -> [w408 w431]
            tunnel: [w405 w430] -> w390
            tunnel: w388 -> [_ w429]
            tunnel: w384 -> [w401 _]
            frame No Error {
              n149 = call "PH_Cam_BaseClass.get data to modify.vi"("i ref in"=w407, "error in (no error)"=w408) -> ("i ref out"=w404:refnum<vi>, "i attribute"=w402:T4, "timed out"=w400:bool, "error out"=w406:errorcluster)  [unwired: 14 in]
              n150 = case shown="False" w400 {
                tunnel: w406 -> [w412 w427]
                tunnel: [w421 w427] -> w405
                tunnel: w404 -> [w420 w428]
                tunnel: [w419 w428] -> w403
                tunnel: w402 -> [w417 _]
                tunnel: w401 -> [w410 _]
                frame False {
                  n151 = Unbundle By Name(w417) -> ("Gui Refs.Histogram"=w409:refnum<vi>, "Gui Refs.Get Histogram"=w413:refnum<vi>)
                  n152 = call "PH_GUI.set boolean GUI object.vi"("Boolean Knob GUI Ref"=w413, "Value"=w410, "error in (no error)"=w412) -> ("error out"=w411:errorcluster)  [unwired: 16 in]
                  n153 = Not A Number/Path/Refnum?(number/path/refnum=w409) -> (NaN/Path/Refnum?=w416:bool)
                  n154 = case shown="False" w416 {
                    tunnel: w411 -> [w425 w426]
                    tunnel: [w424 w426] -> w415
                    tunnel: w409 -> [w423 _]
                    tunnel: u32[] [] ("Value") -> [w422 _]
                    frame False {
                      n155 = property class="WFGraph (strict)"(reference=w423, error in=w425, "Value"=w422) -> (error out=w424:errorcluster)  [unwired: 1 out]
                    }
                    frame True {
                    }
                  }
                  n156 = Bundle By Name(cluster=w417, "Histogram.on"=w410) -> (w418:T4)
                  n157 = call "PH_Cam_BaseClass.set modified data.vi"("i ref in"=w420, "i attribute"=w418, "error in (no error)"=w415) -> ("i ref out"=w419:refnum<vi>, "error out"=w421:errorcluster)  [unwired: 15 in]
                }
                frame True {
                }
              }
            }
            frame Error {
              n158 = call "CoreLib.set data type mismatch.vi"("error in (no error)"=w431, "error source"=w429) -> ("error out"=w430:errorcluster)  [unwired: 17 in]
            }
          }
          n159 = call "BaseProcess.set event status.vi"("i ref in"=w391, "EventStatus"=w388, "error in (no error)"=w390) -> ("i ref out"=w387:refnum<vi>, "error out"=w389:errorcluster)  [unwired: 14 in, 1 out]
          n160 = Unbundle By Name(w389) -> ("code"=w394:i32)
          n161 = case shown="Error" w389 {
            selector: w389 -> [_ w399]
            tunnel: [_ w397] -> w382
            frame No Error {
              (unwired) "" ("source")
            }
            frame Error {
              n162 = Unbundle By Name(w399) -> ("source"=w398:string)
              n163 = call-poly "CoreLib.data 2 byte array.vi"("string"=w398) -> ("byteArray out"=w397:T1)  [unwired: 18 in]
            }
          }
          n164 = Bundle By Name(cluster=w393, "Data"=w382, "Error #"=w394) -> (w392:T2)
        }
        frame "SetMapping" {
          n165 = Unbundle By Name(w444) -> ("Data"=w436:T1)
          n166 = call-poly "CoreLib.byte array 2 data.vi"("byteArray"=w436) -> ("i16"=w437:i16, "error out"=w434:errorcluster)  [unwired: 16 in, 1 out]
          n167 = Not Equal To 0?(x=w437) -> (x != 0?=w435:bool)
          n168 = case shown="No Error" w434 {
            tunnel: [w454 w485] -> w442
            tunnel: w447 -> [w458 w485]
            tunnel: w446 -> [w459 w484]
            tunnel: [w456 w483] -> w441
            tunnel: w439 -> [_ w482]
            tunnel: w435 -> [w452 _]
            frame No Error {
              n169 = call "PH_Cam_BaseClass.get data to modify.vi"("i ref in"=w458, "error in (no error)"=w459) -> ("i ref out"=w455:refnum<vi>, "i attribute"=w453:T4, "timed out"=w451:bool, "error out"=w457:errorcluster)  [unwired: 14 in]
              n170 = case shown="False" w451 {
                tunnel: w457 -> [w462 w480]
                tunnel: [w474 w480] -> w456
                tunnel: w455 -> [w473 w481]
                tunnel: [w472 w481] -> w454
                tunnel: w453 -> [w470 _]
                tunnel: w452 -> [w460 _]
                frame False {
                  n171 = Unbundle By Name(w470) -> ("Gui Refs.Histogram"=w468:refnum<vi>, "Gui Refs.Mapping"=w463:refnum<vi>)
                  n172 = call "PH_GUI.set boolean GUI object.vi"("Boolean Knob GUI Ref"=w463, "Value"=w460, "error in (no error)"=w462) -> ("error out"=w461:errorcluster)  [unwired: 16 in]
                  n173 = Select(t=u8 1 ("Y Scale.Mapping Mode"), s=w460, f=u8 0) -> (s? t:f=w464:u8)
                  n174 = Not A Number/Path/Refnum?(number/path/refnum=w468) -> (NaN/Path/Refnum?=w467:bool)
                  n175 = case shown="False" w467 {
                    tunnel: w461 -> [w478 w479]
                    tunnel: [w477 w479] -> w469
                    tunnel: w468 -> [w476 _]
                    tunnel: w464 -> [w475 _]
                    frame False {
                      n176 = property class="WFGraph (strict)"(reference=w476, error in=w478, "Y Scale.Mapping Mode"=w475) -> (error out=w477:errorcluster)  [unwired: 1 out]
                    }
                    frame True {
                    }
                  }
                  n177 = Bundle By Name(cluster=w470, "Histogram.Mapping"=w460) -> (w471:T4)
                  n178 = call "PH_Cam_BaseClass.set modified data.vi"("i ref in"=w473, "i attribute"=w471, "error in (no error)"=w469) -> ("i ref out"=w472:refnum<vi>, "error out"=w474:errorcluster)  [unwired: 15 in]
                }
                frame True {
                }
              }
            }
            frame Error {
              n179 = call "CoreLib.set data type mismatch.vi"("error in (no error)"=w484, "error source"=w482) -> ("error out"=w483:errorcluster)  [unwired: 17 in]
            }
          }
          n180 = call "BaseProcess.set event status.vi"("i ref in"=w442, "EventStatus"=w439, "error in (no error)"=w441) -> ("i ref out"=w438:refnum<vi>, "error out"=w440:errorcluster)  [unwired: 14 in, 1 out]
          n181 = Unbundle By Name(w440) -> ("code"=w445:i32)
          n182 = case shown="Error" w440 {
            selector: w440 -> [_ w450]
            tunnel: [_ w448] -> w433
            frame No Error {
              (unwired) "" ("source")
            }
            frame Error {
              n183 = Unbundle By Name(w450) -> ("source"=w449:string)
              n184 = call-poly "CoreLib.data 2 byte array.vi"("string"=w449) -> ("byteArray out"=w448:T1)  [unwired: 18 in]
            }
          }
          n185 = Bundle By Name(cluster=w444, "Data"=w433, "Error #"=w445) -> (w443:T2)
        }
        frame "GetFrameRate" {
          n186 = Unbundle By Name(w497) -> ("Data"=w489:T1)
          n187 = call-poly "CoreLib.byte array 2 data.vi"("byteArray"=w489) -> ("i16"=w490:i16, "error out"=w487:errorcluster)  [unwired: 16 in, 1 out]
          n188 = Not Equal To 0?(x=w490) -> (x != 0?=w488:bool)
          n189 = case shown="No Error" w487 {
            tunnel: [w505 w512] -> w495
            tunnel: w500 -> [w507 w512]
            tunnel: w499 -> [w508 w511]
            tunnel: [w506 w510] -> w494
            tunnel: w492 -> [_ w509]
            tunnel: w488 -> [w504 _]
            frame No Error {
              n190 = call "PH_Cam_BaseClass.PC get Frame Rate.vi"("i ref in"=w507, "on"=w504, "error in (no error)"=w508) -> ("i ref out"=w505:refnum<vi>, "error out"=w506:errorcluster)  [unwired: 15 in]
            }
            frame Error {
              n191 = call "CoreLib.set data type mismatch.vi"("error in (no error)"=w511, "error source"=w509) -> ("error out"=w510:errorcluster)  [unwired: 17 in]
            }
          }
          n192 = call "BaseProcess.set event status.vi"("i ref in"=w495, "EventStatus"=w492, "error in (no error)"=w494) -> ("i ref out"=w491:refnum<vi>, "error out"=w493:errorcluster)  [unwired: 14 in, 1 out]
          n193 = Unbundle By Name(w493) -> ("code"=w498:i32)
          n194 = case shown="Error" w493 {
            selector: w493 -> [_ w503]
            tunnel: [_ w501] -> w486
            frame No Error {
              (unwired) "" ("source")
            }
            frame Error {
              n195 = Unbundle By Name(w503) -> ("source"=w502:string)
              n196 = call-poly "CoreLib.data 2 byte array.vi"("string"=w502) -> ("byteArray out"=w501:T1)  [unwired: 18 in]
            }
          }
          n197 = Bundle By Name(cluster=w497, "Data"=w486, "Error #"=w498) -> (w496:T2)
        }
        frame "Connect" {
          n198 = Unbundle By Name(w516) -> ("Data"=w521:T1)
          n199 = call-poly "CoreLib.byte array 2 data.vi"("byteArray"=w521) -> ("string"=w520:string, "error out"=w519:errorcluster)  [unwired: 16 in, 1 out]
          n200 = case shown="No Error" w519 {
            tunnel: [w529 w548] -> w515
            tunnel: w518 -> [w534 w548]
            tunnel: w517 -> [w535 w547]
            tunnel: [w528 w546] -> w514
            tunnel: w513 -> [_ w545]
            tunnel: w520 -> [w527 _]
            frame No Error {
              n201 = call "PH_Cam_BaseClass.get data to modify.vi"("i ref in"=w534, "error in (no error)"=w535) -> ("i ref out"=w532:refnum<vi>, "i attribute"=w531:T4, "timed out"=w530:bool, "error out"=w533:errorcluster)  [unwired: 14 in]
              n202 = case shown="False" w530 {
                tunnel: w533 -> [w536 w543]
                tunnel: [w542 w543] -> w528
                tunnel: w532 -> [w541 w544]
                tunnel: [w540 w544] -> w529
                tunnel: w531 -> [w538 _]
                tunnel: w527 -> [w537 _]
                frame False {
                  n203 = Bundle By Name(cluster=w538, "Cam.Camera ID"=w537) -> (w539:T4)
                  n204 = call "PH_Cam_BaseClass.set modified data.vi"("i ref in"=w541, "i attribute"=w539, "error in (no error)"=w536) -> ("i ref out"=w540:refnum<vi>, "error out"=w542:errorcluster)  [unwired: 15 in]
                }
                frame True {
                }
              }
            }
            frame Error {
              n205 = call "CoreLib.set data type mismatch.vi"("error in (no error)"=w547, "error source"=w545) -> ("error out"=w546:errorcluster)  [unwired: 17 in]
            }
          }
          n206 = call "BaseProcess.set event status.vi"("i ref in"=w515, "EventStatus"=w513, "error in (no error)"=w514) -> ("i ref out"=w523:refnum<vi>, "error out"=w524:errorcluster)  [unwired: 14 in, 1 out]
          n207 = Unbundle By Name(w524) -> ("code"=w526:i32)
          n208 = case shown="Error" w524 {
            selector: w524 -> [_ w551]
            tunnel: [_ w549] -> w522
            frame No Error {
              (unwired) "" ("source")
            }
            frame Error {
              n209 = Unbundle By Name(w551) -> ("source"=w550:string)
              n210 = call-poly "CoreLib.data 2 byte array.vi"("string"=w550) -> ("byteArray out"=w549:T1)  [unwired: 18 in]
            }
          }
          n211 = Bundle By Name(cluster=w516, "Data"=w522, "Error #"=w526) -> (w525:T2)
        }
      }
    }
    frame Error {
    }
  }
  "answer cluster" <- w7
  "i ref out" <- w4
  "error out" <- w3
